vi "Build Bookmark Manager.vi"(5 "Project File":path, 7 "Target Version":string="15.0", 8 "Error In":errorcluster) -> (0 "Error Out":errorcluster)   [LabVIEW 2017]
uses:
  <vilib>/AppBuilder/AB_API_Simple/Build (path).vi
  <vilib>/AppBuilder/AB_API_Simple/NI_App_Builder_API.lvlib
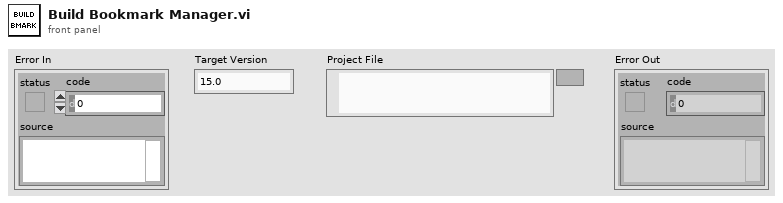
[diagram p1: front panel]
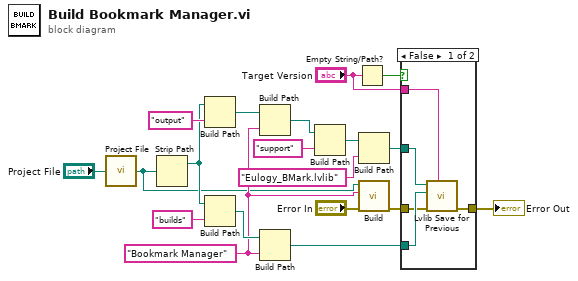
[diagram p0: block diagram]
diagram:
  w9 = "Bookmark Manager" ("name or relative path")
  n1 = call "Project File.vi"("Project File In"="Project File") -> ("Project File Out"=w1:path)
  n2 = Strip Path(path=w1) -> (stripped path=w4:path)  [unwired: 1 out]
  n3 = Build Path(base path=w4, name or relative path="output") -> (appended path=w18:path)
  n4 = Build Path(base path=w4, name or relative path="builds") -> (appended path=w11:path)
  n5 = Build Path(base path=w18, name or relative path=w9) -> (appended path=w17:path)
  n6 = Build Path(base path=w11, name or relative path=w9) -> (appended path=w10:path)
  n7 = Build Path(base path=w17, name or relative path="support") -> (appended path=w15:path)
  n8 = Empty String/Path?(string/path="Target Version") -> (empty?=w2:bool)
  n9 = Build Path(base path=w15, name or relative path="Eulogy_BMark.lvlib") -> (appended path=w13:path)
  n10 = call-poly <vilib>:"Build.vi"("error in (no error)"="Error In", "Name of build specification (if empty: build all)"=w9, "Path to project"=w1) -> ("error out"=w8:errorcluster)  [unwired: 7 in, 1 out]
  n11 = case shown="False" w2 {
    tunnel: w13 -> [w24 _]
    tunnel: w10 -> [w23 _]
    tunnel: w8 -> [w22 w25]
    tunnel: [w21 w25] -> w6
    tunnel: "Target Version" -> [w20 _]
    frame False {
      n12 = call "Lvlib Save for Previous.vi"("Target Version"=w20, "Error In"=w22, "Destination Folder"=w23, "Original lvlib"=w24) -> ("Error Out"=w21:errorcluster)  [unwired: 7 in]
    }
    frame True {
    }
  }
  "Error Out" <- w6
